vi "Panel.vi"(10 "Actor":refnum<class "Actor.lvclass">, 11 "Dev Actor Panel":refnum<class "Dev Actor Panel.lvclass">) -> ()   [LabVIEW 2021, in "Dev Actor Panel.lvclass"]
uses:
  Dev Actor Panel.lvclass
  <vilib>/jettl/jettl/Actor/Actor/Actor.lvclass
  Dev Actor Panel.lvclass/Dev Actor Panel.ctl
  <vilib>/jettl/jettl/Actor/Msgs/Destroy/Destroy Msg/Destroy Msg.lvclass
  C:/Program Files/National Instruments/LabVIEW 2021/vi.lib/jettl/jettl/Actor/Msg/Msg.lvclass
  Pop Up/Pop Up Msg/Pop Up Msg.lvclass
panel:
  in  "Pop Up":bool
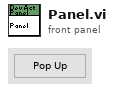
[diagram p1: front panel]
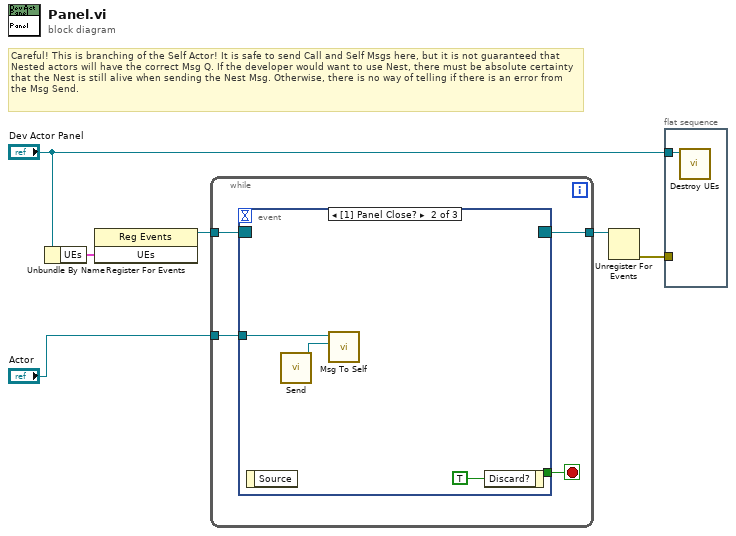
[diagram p0: block diagram]
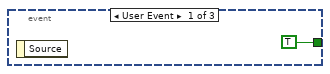
[diagram p2: hidden frame]
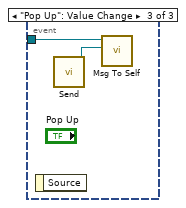
[diagram p3: hidden frame]
diagram:
  # "Careful! This is branching of the Self Actor! It is safe to send Call and Self Msgs here, but it is not guaranteed that Nested actors will have the correct Msg Q. If the developer would want to use Nest, there must be absolute certainty that the Nest is still alive when sending the Nest Msg. Otherwise, there is no way of telling if there is an error from the Msg Send."
  n1 = Unbundle By Name("Dev Actor Panel") -> ("UEs"=w3:cluster{"Teardown":refnum<user-event>})
  n2 = register-events ("Main Register for Events")(w3) -> (reference out=w4:refnum<event-registration>)  [unwired: 2 in, 1 out]
  n3 = while {
    tunnel: w4 -> [w10]
    tunnel: [w8] -> w5
    tunnel: "Actor" -> [w7]
    stop <- w9 stop-if-true
    n4 = event "UI Events" shown="[1] Panel Close?" {
      selector: w10 -> [_ _ _]
      dyn-events: [_ _ _] -> w8
      timeout: _ -> [_ _ _]
      tunnel: [TRUE _ _] -> w9
      tunnel: w7 -> [_ w13 w15]
      event User Event {
        n5 = event-data() -> ()  [unwired: 1 in, 1 out]
      }
      event Panel Close? {
        n6 = event-data() -> ()  [unwired: 1 in, 1 out]
        n7 = call <vilib>:"Send.vi"() -> ("Destroy Msg out"=w12:refnum<class "Destroy Msg.lvclass">)  [unwired: 11 in]
        n8 = call-dynamic "Msg To Self.vi"("Msg"=w12, "Actor in"=w13) -> ()  [unwired: 9 in, 1 out]
        n9 = event-data("Discard?"=TRUE) -> ()  [unwired: 1 in, 1 out]
      }
      event "Pop Up": Value Change {
        n10 = event-data() -> ()  [unwired: 1 in, 1 out]
        n11 = call <vilib>:"Send.vi"() -> ("Pop Up Msg out"=w16:refnum<class "Pop Up Msg.lvclass">)  [unwired: 11 in]
        n12 = call-dynamic "Msg To Self.vi"("Msg"=w16, "Actor in"=w15) -> ()  [unwired: 9 in, 1 out]
      }
    }
  }
  n13 = Unregister For Events(event registration refnum=w5) -> (error out=w2:errorcluster)  [unwired: 1 in]
  n14 = flat-sequence {
    tunnel: "Dev Actor Panel" -> [w17]
    tunnel: w2 -> [_]
    frame #0 {
      n15 = call-dynamic "Destroy UEs.vi"("Dev Actor Panel in"=w17) -> ()  [unwired: 10 in, 1 out]
    }
  }
